vi "alarm map.vi"(8 "error in (no error)":errorcluster, 11 "map in":T2) -> (0 "error out":errorcluster, 2 "change?":bool, 3 "map out":T1)   [LabVIEW 2016, in "Alarm interface.lvlib"]
uses:
  Alarm interface.lvlib
  <vilib>/xml/Load XML File.vi
  <vilib>/xml/Close Reference(Node).vi
  <vilib>/xml/NI_XML.lvlib
  <resource>/objmgr/DOMUserDefRef.rc
panel:
  out "XML":string
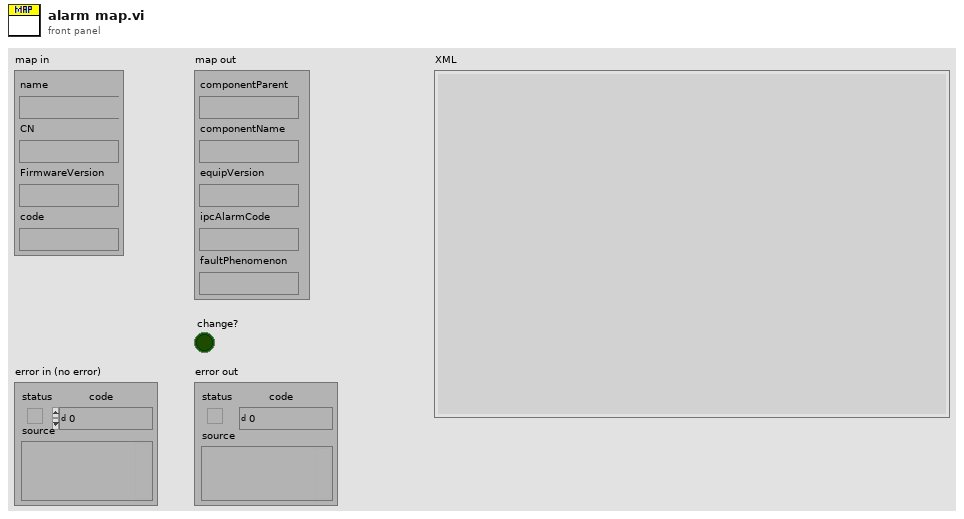
[diagram p1: front panel]
types:
  T1 = typedef "Alarm interface.lvlib/map out.ctl" = cluster{"componentParent":string, "componentName":string, "equipVersion":string, "ipcAlarmCode":string, "faultPhenomenon":string}
  T2 = typedef "Alarm interface.lvlib/map in.ctl" = cluster{"name":string, "CN":string, "FirmwareVersion":string, "code":string}
  T3 = cluster{"name":bool, "CN":bool, "FirmwareVersion":bool, "code":bool}
  T4 = cluster{"[0]":string, "[1]":string, "[2]":string, "[3]":string, "[4]":string}
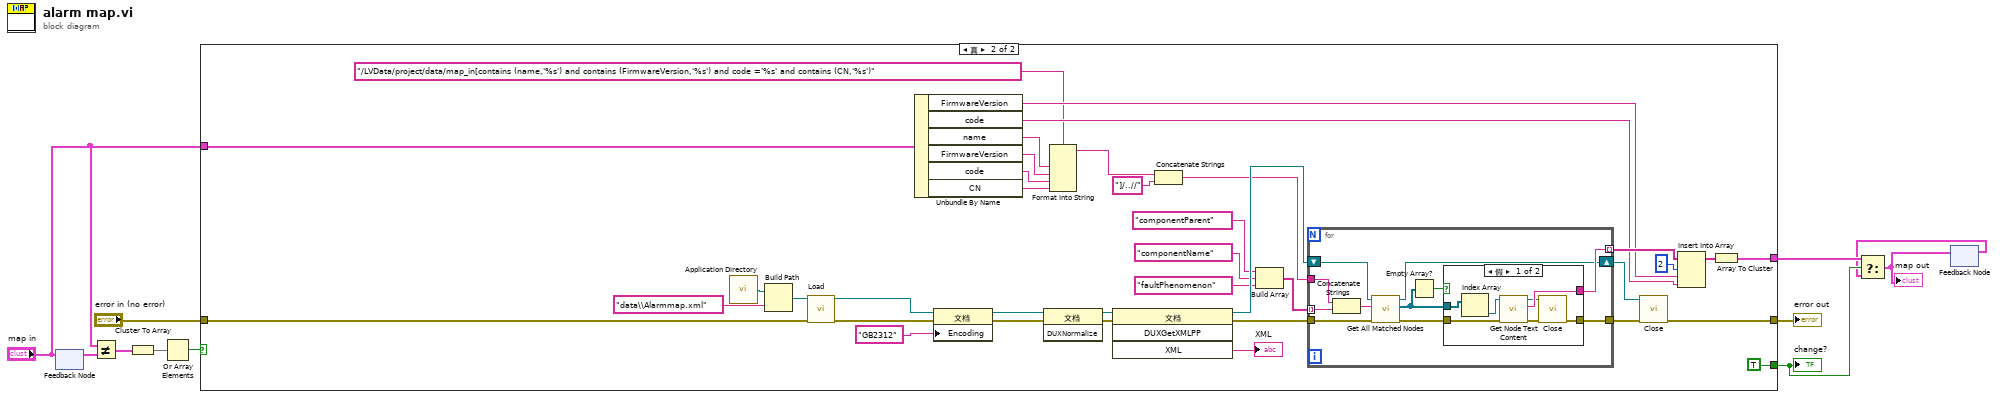
[diagram p0: block diagram]
diagram:
  n1 = feedback-in #1("map in") -> ()
  n2 = feedback #1() -> (w8:T2)  [unwired: 1 in]
  n3 = Not Equal?(x="map in", y=w8) -> (x != y?=w7:T3)
  n4 = Cluster To Array(cluster=w7) -> (array=w6:bool[])
  n5 = Or Array Elements(Boolean array=w6) -> (logical OR=w5:bool)
  n6 = case shown="真" w5 {
    tunnel: [_ w48] -> w3
    tunnel: [_ w47] -> w11
    tunnel: "error in (no error)" -> [_ w46]
    tunnel: "map in" -> [_ w45]
    tunnel: [_ TRUE] -> w4
    frame False {
    }
    frame True {
      n7 = call <vilib>:"Application Directory.vi"() -> ("Application Directory"=w31:path)
      n8 = Build Path(base path=w31, name or relative path="data\\Alarmmap.xml" ("字符串")) -> (appended path=w29:path)
      n9 = call-poly <vilib>:"Load.vi"("path to XML document"=w29, "error in (no error)"=w46) -> ("DOM document out"=w41:refnum<k20>, "error out"=w40:errorcluster)  [unwired: 11 in, 1 out]
      n10 = Unbundle By Name(w45) -> ("FirmwareVersion"=w17:string, "code"=w16:string, "name"=w23:string, "FirmwareVersion"=w32:string, "code"=w18:string, "CN"=w14:string)
      n11 = property on="属性节点" class="文档"(reference=w41, error in=w40, "Encoding"="GB2312" ("文档编码")) -> (reference out=w43:refnum<k20>, error out=w42:errorcluster)
      n12 = invoke on="调用节点" class="文档" method="DUXNormalize"(reference=w43, error in=w42) -> (reference out=w39:refnum<k20>, error out=w38:errorcluster)  [unwired: 1 in, 1 out]
      n13 = Format Into String(format string="/LVData/project/data/map_in[contains (name,'%s') and contains (FirmwareVersion,'%s') and code ='%s' and contains (CN,'%s')" ("字符串"), w23, w32, w18, w14) -> (resulting string=w28:string)  [unwired: 2 in, 1 out]
      n14 = invoke on="调用节点" class="文档" method="DUXGetXMLPP"(reference=w39, error in=w38) -> (reference out=w37:refnum<k20>, error out=w33:errorcluster, "XML"=→"XML":string)  [unwired: 2 in, 1 out]
      n15 = Concatenate Strings(w28, "]/..//" ("字符串")) -> (w34:string)
      n16 = Build Array("componentParent", "componentName", "faultPhenomenon") -> (w36:string[])
      n17 = for {
        tunnel: w34 -> [w55]
        tunnel: w36 -> [w54] mode=indexing
        tunnel: [w58] -> w20 mode=indexing
        tunnel: [w51] -> w25
        tunnel: w33 -> [w53]
        shift-right: [w57] -> w26
        shift-left: w37 -> [w59]
        n18 = Concatenate Strings(w55, w54) -> (w52:string)
        n19 = call <vilib>:"Get All Matched Nodes.vi"("error in (no error)"=w53, "XPath expression"=w52, "node in"=w59) -> ("error out"=w56:errorcluster, "node result array"=w49:refnum<k20>[], "node out"=w57:refnum<k20>)  [unwired: 6 in]
        n20 = Empty Array?(array=w49) -> (empty?=w50:bool)
        n21 = case shown="假" w50 {
          tunnel: [w66 _] -> w58
          tunnel: w56 -> [w65 w67]
          tunnel: [w62 w67] -> w51
          tunnel: w49 -> [w61 _]
          frame False {
            n22 = Index Array(array=w61) -> (element=w60:refnum<k20>)  [unwired: 1 in]
            n23 = call <vilib>:"Get Node Text Content.vi"("error in (no error)"=w65, "node in"=w60) -> ("error out"=w63:errorcluster, "node text"=w66:string, "node out"=w64:refnum<k20>)  [unwired: 7 in]
            n24 = call-poly <vilib>:"Close.vi"("error in (no error)"=w63, "node"=w64) -> ("error out"=w62:errorcluster)  [unwired: 7 out]
          }
          frame True {
          }
        }
      }
      n25 = call-poly <vilib>:"Close.vi"("error in (no error)"=w25, "node"=w26) -> ("error out"=w47:errorcluster)  [unwired: 7 out]
      n26 = Insert Into Array(array=w20, index=2 ("索引"), new element #1=w17, new element #2=w16) -> (w21:string[])
      n27 = Array To Cluster(array=w21) -> (cluster=w48:T4)
    }
  }
  "error out" <- w11
  "change?" <- w4
  n28 = feedback #2() -> (w1:T4)  [unwired: 1 in]
  n29 = Select(t=w3, s=w4, f=w1) -> (s? t:f=w2:T4)
  "map out" <- w2
  n30 = feedback-in #2(w2) -> ()
